vi "Push Error if Different.vi"(0 "Error Queue":refnum<queue>, 11 "error in":errorcluster) -> ()   [LabVIEW 2013, in "AIT 664 Custom Device.lvlib"]
doc: "Transmit errors from async vi back to pcl."
uses:
  AIT 664 Custom Device.lvlib
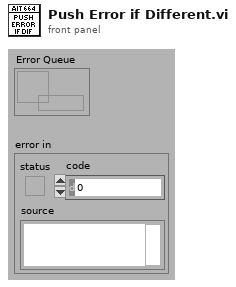
[diagram p1: front panel]
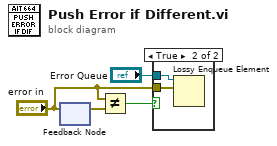
[diagram p0: block diagram]
diagram:
  n1 = feedback #1() -> (w1:errorcluster)  [unwired: 1 in]
  n2 = feedback-in #1("error in") -> ()
  n3 = Not Equal?(x="error in", y=w1) -> (x != y?=w3:bool)
  n4 = case shown="True" w3 {
    tunnel: "error in" -> [_ w6]
    tunnel: "Error Queue" -> [_ w5]
    frame False {
    }
    frame True {
      n5 = Lossy Enqueue Element(queue=w5, element=w6) -> ()  [unwired: 1 in, 4 out]
    }
  }
